vi "Anritsu VNA Preset.vi"(7 "Anritsu VNA":T1, 8 "error in (no error)":errorcluster, 11 "VISA Resource Name":refnum<visa-resource-name>) -> (0 "error out":errorcluster, 3 "dup VISA Resource Name":refnum<visa-resource-name>)   [LabVIEW 2011]
uses:
  TypeDefs/Anritsu VNA Instrument Info.ctl
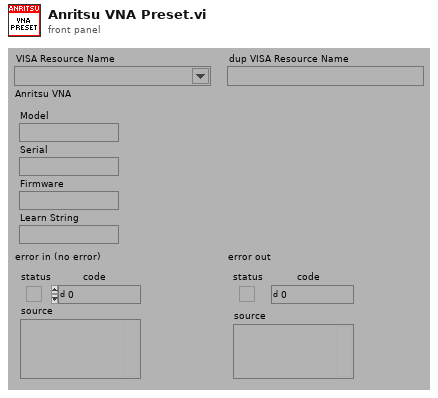
[diagram p1: front panel]
types:
  T1 = typedef "Anritsu VNA Instrument Info.ctl" = cluster{"Model":string, "Serial":string, "Firmware":string, "Learn String":string}
  T2 = typedef "Anritsu VNA Model.ctl" = enum16{"Not Supported", "37XXXX", "MS20XXX", "MS462XX", "MS464XX"}
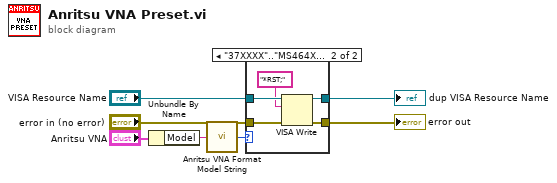
[diagram p0: block diagram]
diagram:
  n1 = Unbundle By Name("Anritsu VNA") -> ("Model"=w2:string)
  n2 = call "Anritsu VNA Format Model String.vi"("Model"=w2) -> ("Model"=w1:T2)
  n3 = case shown="\"37XXXX\"..\"MS464XX\"" w1 {
    tunnel: "error in (no error)" -> [w8 w14]
    tunnel: "VISA Resource Name" -> [w9 w13]
    tunnel: [w9 w12] -> w5
    tunnel: [w8 w11] -> w4
    frame "Not Supported" {
    }
    frame "37XXXX".."MS464XX" {
      n4 = VISA Write(VISA resource name=w13, write buffer="*RST;", error in (no error)=w14) -> (VISA resource name out=w12:refnum<visa-resource-name>, error out=w11:errorcluster)  [unwired: 1 out]
    }
  }
  "error out" <- w4
  "dup VISA Resource Name" <- w5
